vi "email sender.vi"(7 "Body":string="It works!", 8 "error in (no error)":errorcluster, 9 "Subject":string="Sending TLS Authenticated Email", 10 "Recipient's Name":string="Jane Doe", 11 "Recipient's Email Address Address":string) -> (0 "error out":errorcluster)   [LabVIEW 2012]
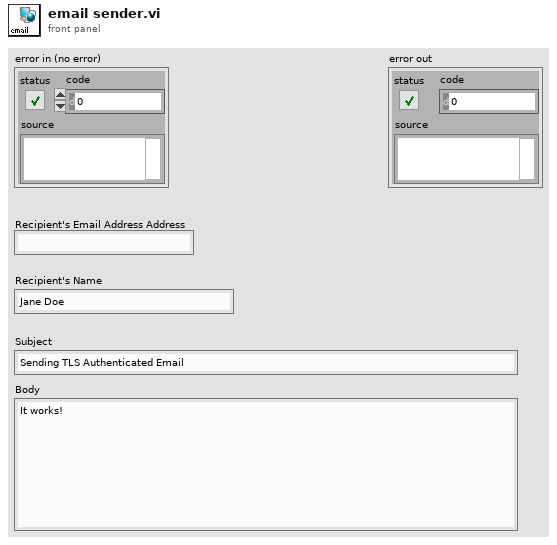
[diagram p1: front panel]
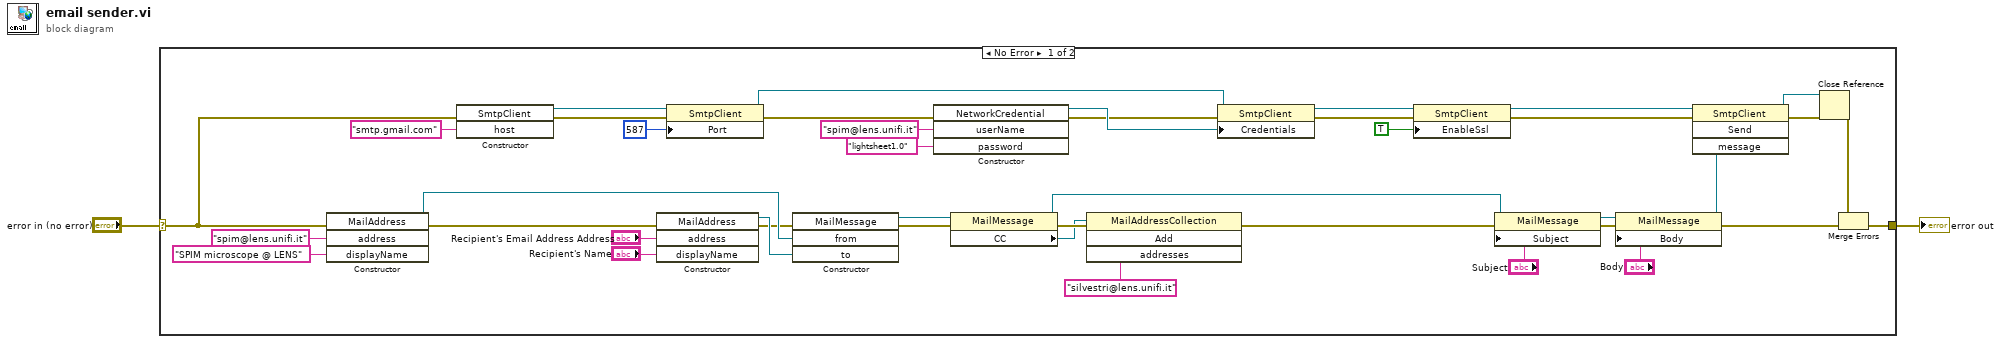
[diagram p0: block diagram]
diagram:
  n1 = case shown="No Error" "error in (no error)" {
    selector: "error in (no error)" -> [w11 w44]
    tunnel: [w4 w44] -> w1
    frame No Error {
      n2 = constructor class="MailAddress"(error in=w11, "address"="spim@lens.unifi.it" ("Sender's Email Address (eg: jsmith77@gmail.com)"), "displayName"="SPIM microscope @ LENS" ("Sender's Name")) -> (reference out=w42:refnum<k24>, error out=w13:errorcluster)  [unwired: 2 in, 3 out]
      n3 = constructor class="SmtpClient"(error in=w11, "host"="smtp.gmail.com" ("Outgoing Mail Server (SMTP)")) -> (reference out=w27:refnum<k24>, error out=w23:errorcluster)  [unwired: 2 in, 2 out]
      n4 = constructor class="MailAddress"(error in=w13, "address"="Recipient's Email Address Address", "displayName"="Recipient's Name") -> (reference out=w43:refnum<k24>, error out=w12:errorcluster)  [unwired: 2 in, 3 out]
      n5 = property class="SmtpClient"(reference=w27, error in=w23, "Port"=587) -> (reference out=w26:refnum<k24>, error out=w10:errorcluster)
      n6 = constructor class="MailMessage"(error in=w12, "from"=w42, "to"=w43) -> (reference out=w18:refnum<k24>, error out=w17:errorcluster)  [unwired: 2 in, 3 out]
      n7 = constructor class="NetworkCredential"(error in=w10, "userName"="spim@lens.unifi.it" ("GMAIL Account User ID (eg: jsmity77)"), "password"="lightsheet1.0" ("GMAIL Account Password")) -> (reference out=w28:refnum<k24>, error out=w9:errorcluster)  [unwired: 2 in, 3 out]
      n8 = property class="MailMessage"(reference=w18, error in=w17) -> (reference out=w16:refnum<k24>, error out=w8:errorcluster, "CC"=w7:refnum<k24>)
      n9 = invoke class="MailAddressCollection" method="Add"(reference=w7, error in=w8, "addresses"="silvestri@lens.unifi.it" ("CC (Carbon Copy Recipient - Optional)")) -> (error out=w3:errorcluster)  [unwired: 1 in, 3 out]
      n10 = property class="SmtpClient"(reference=w26, error in=w9, "Credentials"=w28) -> (reference out=w25:refnum<k24>, error out=w22:errorcluster)
      n11 = property class="SmtpClient"(reference=w25, error in=w22, "EnableSsl"=TRUE ("Enable SSL")) -> (reference out=w24:refnum<k24>, error out=w21:errorcluster)
      n12 = property class="MailMessage"(reference=w16, error in=w3, "Subject"="Subject") -> (reference out=w33:refnum<k24>, error out=w41:errorcluster)
      n13 = property class="MailMessage"(reference=w33, error in=w41, "Body"="Body") -> (reference out=w20:refnum<k24>, error out=w5:errorcluster)
      n14 = invoke class="SmtpClient" method="Send"(reference=w24, error in=w21, "message"=w20) -> (reference out=w15:refnum<k24>, error out=w14:errorcluster)  [unwired: 1 in, 2 out]
      n15 = Close Reference(reference=w15, error in (no error)=w14) -> (error out=w6:errorcluster)
      n16 = Merge Errors(w6, w5) -> (w4:errorcluster)
    }
    frame Error {
    }
  }
  "error out" <- w1
